vi "init_hw.vi"(8 "error in (no error)":errorcluster, 11 "glaz in":refnum<class "glaz.lvclass">) -> (0 "error out":errorcluster, 2 "success ?":bool=TRUE, 3 "glaz out":refnum<class "glaz.lvclass">)   [LabVIEW 2019, in "glaz.lvlib" / "glaz.lvclass"]
uses:
  glaz.lvclass
  C:/Users/lars/Desktop/TransientAbsorptionDAQ/_camera/_camera.lvlibp/_cameraClass/_camera.lvclass
  glaz.lvclass/glaz.ctl
  _camera/_camera.lvlibp/_cameraClass/Write camera name and version.vi
panel:
  out "minorVersion":i32
  out "majorVersion":i32
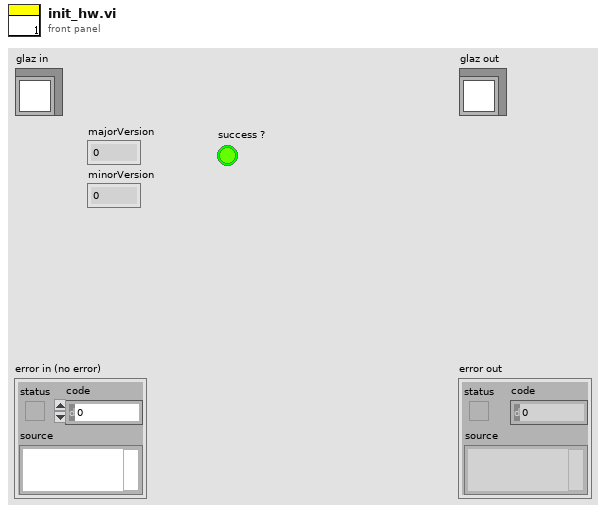
[diagram p1: front panel]
types:
  T1 = enum16{"x1", "x2", "x4", "x8", "x16", "x32", "x64", "x128", "x256"}
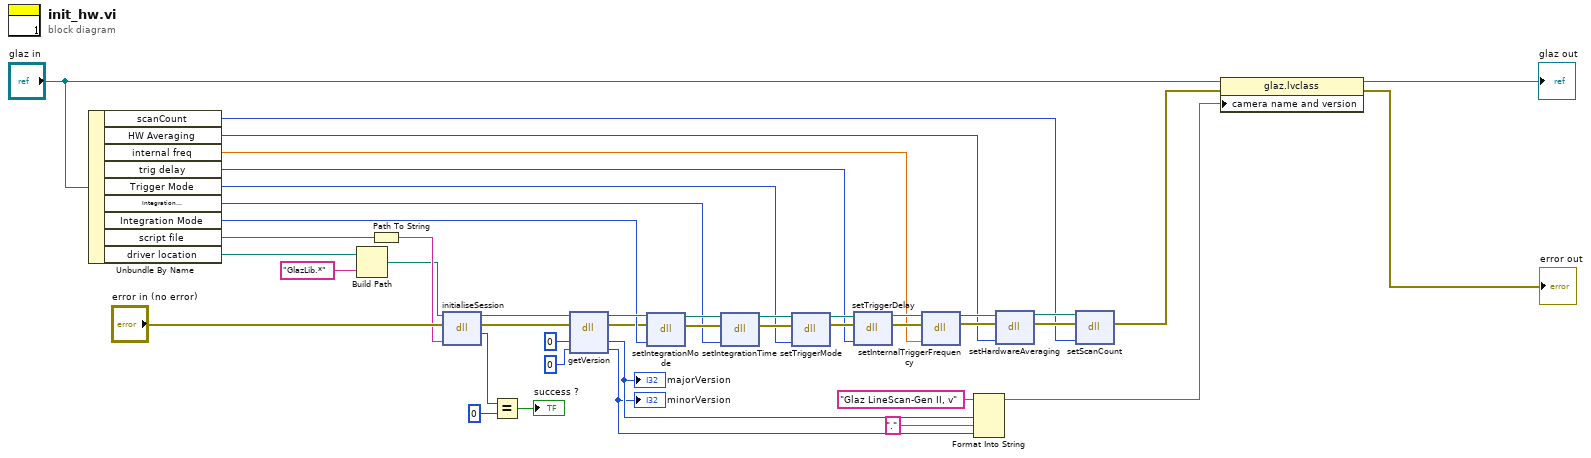
[diagram p0: block diagram]
diagram:
  n1 = Unbundle By Name("glaz in") -> ("scanCount"=w13:i32, "HW Averaging"=w16:T1, "internal freq"=w19:dbl, "trig delay"=w22:i32, "Trigger Mode"=w25:enum16{"External", "Internal", "Burst"}, "Integration\nTime [us]"=w28:i32, "Integration Mode"=w32:enum16{"PulseSync", "TimeFill"}, "script file"=w43:path, "driver location"=w12:path)
  n2 = Build Path(base path=w12, name or relative path="GlazLib.*") -> (appended path=w10:path)
  n3 = Path To String(path=w43) -> (string=w39:string)
  n4 = dll-call lib="C:/Program Files/National Instruments/LabVIEW 2019/user.lib/GlazLabView/GlazLib.*" fn="initialiseSession"(path in=w10, error in="error in (no error)", "scriptFileName"=w39) -> (path out=w34:path, error out=w35:errorcluster, "return type"=w38:i32)  [unwired: 2 in]
  n5 = Equal?(x=w38, y=0) -> (x = y?=→"success ?":bool)
  n6 = dll-call lib="C:/Program Files/National Instruments/LabVIEW 2019/user.lib/GlazLabView/GlazLib.*" fn="getVersion"(path in=w34, error in=w35, "majorVersion"=0, "minorVersion"=0) -> (path out=w33:path, error out=w31:errorcluster, "majorVersion"=w5:i32, "minorVersion"=w2:i32)  [unwired: 2 in]
  "majorVersion" <- w5
  "minorVersion" <- w2
  n7 = dll-call lib="C:/Program Files/National Instruments/LabVIEW 2019/user.lib/GlazLabView/GlazLib.*" fn="setIntegrationMode"(path in=w33, error in=w31, "mode"=w32) -> (path out=w30:path, error out=w29:errorcluster)  [unwired: 3 in]
  n8 = dll-call lib="C:/Program Files/National Instruments/LabVIEW 2019/user.lib/GlazLabView/GlazLib.*" fn="setIntegrationTime"(path in=w30, error in=w29, "us"=w28) -> (path out=w27:path, error out=w26:errorcluster)  [unwired: 3 in]
  n9 = dll-call lib="C:/Program Files/National Instruments/LabVIEW 2019/user.lib/GlazLabView/GlazLib.*" fn="setTriggerMode"(path in=w27, error in=w26, "mode"=w25) -> (path out=w24:path, error out=w23:errorcluster)  [unwired: 3 in]
  n10 = dll-call lib="C:/Program Files/National Instruments/LabVIEW 2019/user.lib/GlazLabView/GlazLib.*" fn="setTriggerDelay"(path in=w24, error in=w23, "us"=w22) -> (path out=w21:path, error out=w20:errorcluster)  [unwired: 3 in]
  n11 = dll-call lib="C:/Program Files/National Instruments/LabVIEW 2019/user.lib/GlazLabView/GlazLib.*" fn="setInternalTriggerFrequency"(path in=w21, error in=w20, "Hz"=w19) -> (path out=w18:path, error out=w17:errorcluster)  [unwired: 3 in]
  n12 = Format Into String(initial string="Glaz LineScan-Gen II, v", w5, ".", w2) -> (resulting string=w1:string)  [unwired: 2 in, 1 out]
  n13 = dll-call lib="C:/Program Files/National Instruments/LabVIEW 2019/user.lib/GlazLabView/GlazLib.*" fn="setHardwareAveraging"(path in=w18, error in=w17, "averaging"=w16) -> (path out=w14:path, error out=w15:errorcluster)  [unwired: 3 in]
  n14 = dll-call lib="C:/Program Files/National Instruments/LabVIEW 2019/user.lib/GlazLabView/GlazLib.*" fn="setScanCount"(path in=w14, error in=w15, "scanCount"=w13) -> (error out=w7:errorcluster)  [unwired: 3 in, 1 out]
  n15 = property class="glaz.lvclass"(reference="glaz in", error in=w7, "camera name and version"=w1) -> (reference out=→"glaz out":refnum<class "glaz.lvclass">, error out=→"error out":errorcluster)
